vi "OCTavion_Main.vi"() -> ()   [LabVIEW 2016]
panel:
  out "Status":T1
  out "OCT En-face / Volume":dbl[][](graph)
  out "OCT B-Scan":dbl[][](graph)
  out "OCT Spectrum":dbl[][](graph)
  out "Camera Image":dbl[][](graph)
  in  "Acquisition title":string
  in  "Path":path
  in  "Settings":T2(tab)
  in  "Preview Button":bool
  in  "Acquire Button":bool
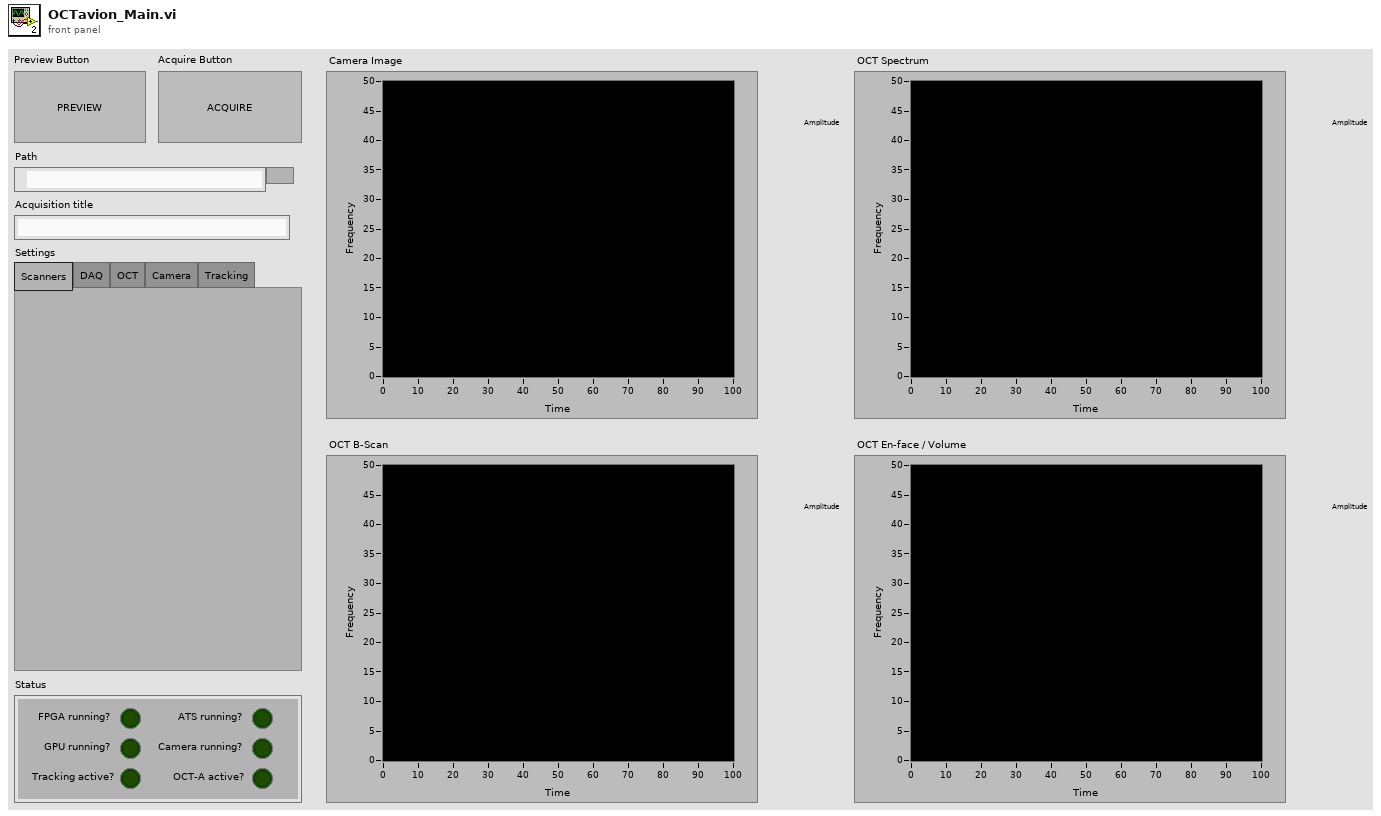
[diagram p1: front panel]
types:
  T1 = cluster{"FPGA running?":bool, "GPU running?":bool, "ATS running?":bool, "Camera running?":bool, "Tracking active?":bool, "OCT-A active?":bool}
  T2 = enum32{"Scanners", "DAQ", "OCT", "Camera", "Tracking"}
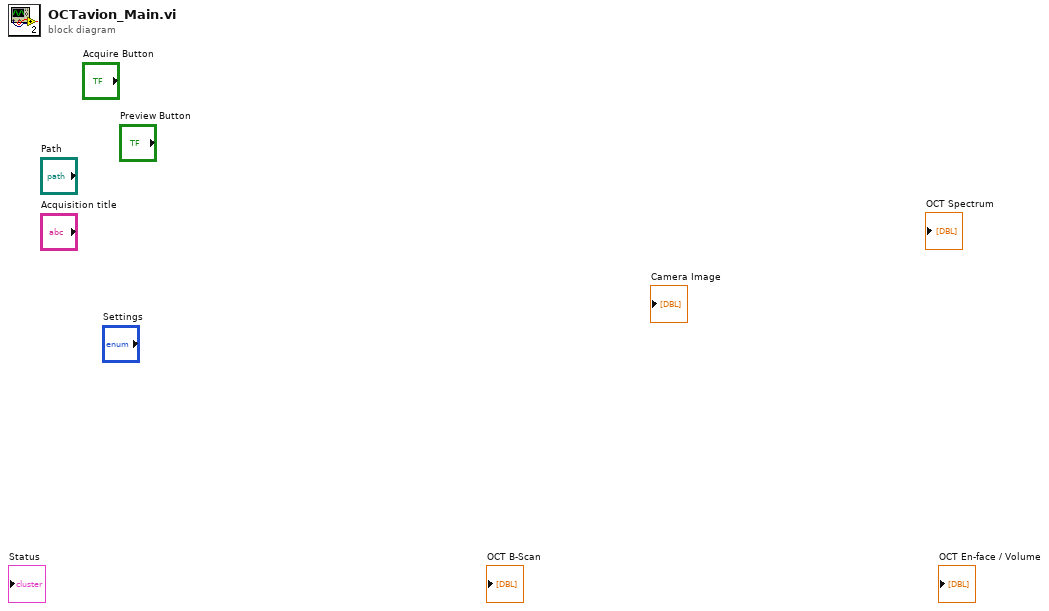
[diagram p0: block diagram]
diagram:
